vi "c_ctre_phoenix6_platform_canbus_get_status.vi"(0 "Numeric 3":sgl, 1 "Numeric 5":u32, 2 "Numeric 7":u32, 3 "Numeric 9":u32, 4 "Numeric 11":u32, 5 "String 2":string, 6 "Numeric 12":u8) -> (20 "Numeric":i32, 21 "Numeric 2":sgl, 22 "Numeric 4":u32, 23 "Numeric 6":u32, 24 "Numeric 8":u32, 25 "Numeric 10":u32, 26 "String":string)   [LabVIEW 2023]
uses:
  <vilib>/Rock Robotics/WPI/ThirdParty/Phoenix-LabVIEW/Controls/DriverLib.ctl
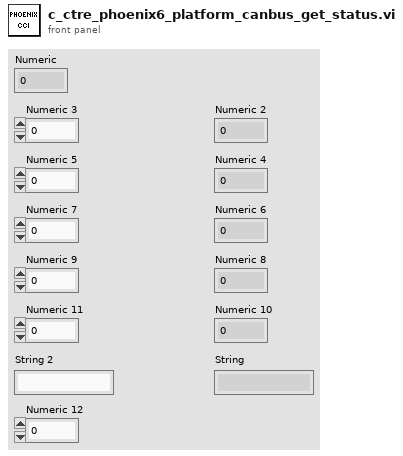
[diagram p1: front panel]
types:
  T1 = typedef "DriverLib.ctl" = path
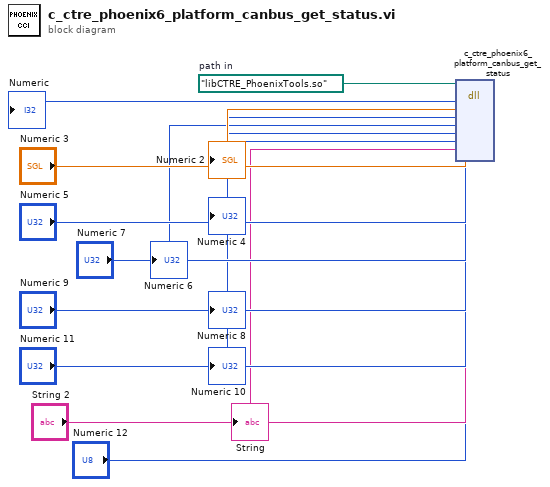
[diagram p0: block diagram]
diagram:
  w15 = T1 path "libCTRE_PhoenixTools.so"  # path in
  n1 = dll-call lib="?" fn="c_ctre_phoenix6_platform_canbus_get_status"(path in=w15, "Numeric 3", "Numeric 5", "Numeric 7", "Numeric 9", "Numeric 11", "String 2", "Numeric 12") -> (→"Numeric":i32, →"Numeric 2":sgl, →"Numeric 4":u32, →"Numeric 6":u32, →"Numeric 8":u32, →"Numeric 10":u32, →"String":string)  [unwired: 3 in, 2 out]
